vi "Rx Message to Transfer Handle - RT.vi"(8 "error in":errorcluster, 9 "message":T2={"name"="", "message type"="BC to RT", "endpoint Tx"={"terminal address"=0, "subaddress"=0}, "endpoint Rx"={"terminal address"=0, "subaddress"=0}, "create timestamp channel"=FALSE, "mode code"=0, "number of words"=0, "parameters"=[]}, 11 "remote terminal handles":u64[](array[numeric])) -> (0 "error out":errorcluster, 2 "valid?":bool, 3 "Rx read info":T1)   [LabVIEW 2020, in "AIM MIL-STD-1553 Engine.lvlib" / "Custom Device.lvlib"]
uses:
  Custom Device.lvlib
  Shared/Message Definition.ctl
  Shared/Message Type.ctl
  Shared/Terminal Endpoint.ctl
  Shared/Address.ctl
  Shared/Parameter Definition.ctl
  Shared/Rx Read Info.ctl
  <instrlib>/BTI1553Lib/Public/Controls/1553 Transfer Direction.ctl
  <instrlib>/BTI1553Lib/Public/Controls/1553 RT Transfer Type.ctl
  <instrlib>/BTI1553Lib/Private/RT/Configure/Get RT Xfer Handle.vi
  <instrlib>/BTI1553Lib/BTI1553LV.lvlib
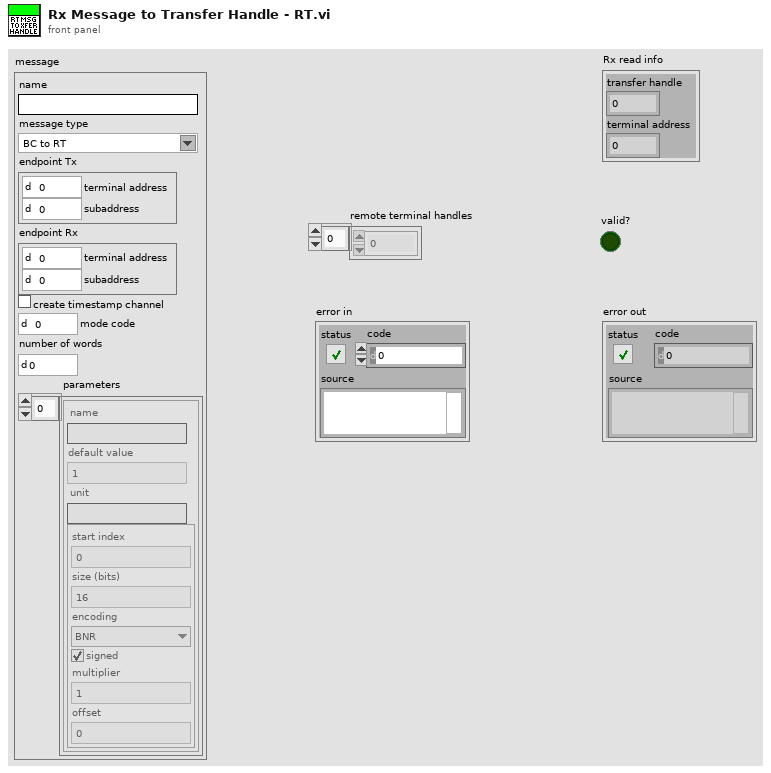
[diagram p1: front panel]
types:
  T1 = typedef "Rx Read Info.ctl" = cluster{"transfer handle":u64, "terminal address":u16}
  T2 = typedef "Message Definition.ctl" = cluster{"name":string, "message type":T3, "endpoint Tx":T4, "endpoint Rx":T4, "create timestamp channel":bool, "mode code":u16, "number of words":u16, "parameters":cluster{"name":string, "default value":dbl, "unit":string, "parameter definition":T6}[]}
  T3 = typedef "Message Type.ctl" = string
  T4 = typedef "Terminal Endpoint.ctl" = cluster{"terminal address":T5, "subaddress":T5}
  T5 = typedef "Address.ctl" = u16
  T6 = typedef "Parameter Definition.ctl" = cluster{"start index":i32, "size (bits)":i32, "encoding":enum16{"BNR", "BCD", "Discrete"}, "signed":bool, "multiplier":dbl, "offset":dbl}
  T7 = typedef "BTI1553LV.lvlib/1553 RT Transfer Type.ctl" = u32
  T8 = typedef "BTI1553LV.lvlib/1553 Transfer Direction.ctl" = u32
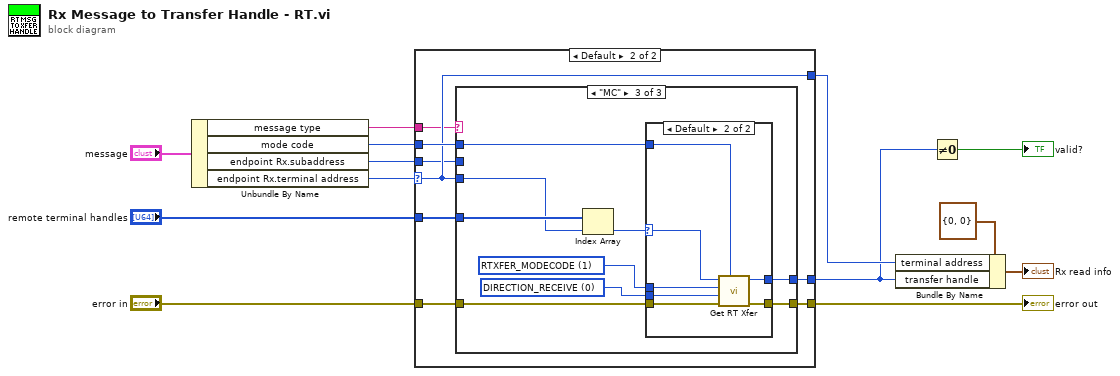
[diagram p0: block diagram]
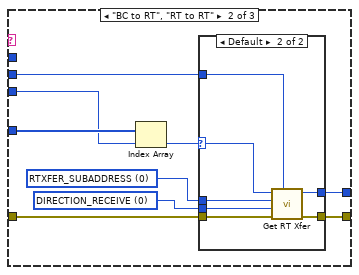
[diagram p4: hidden frame]
diagram:
  n1 = Unbundle By Name("message") -> ("message type"=w2:T3, "mode code"=w11:u16, "endpoint Rx.subaddress"=w1:T5, "endpoint Rx.terminal address"=w13:T5)
  n2 = case shown="Default" w13 {
    selector: w13 -> [_ w17]
    tunnel: "error in" -> [w14 w22]
    tunnel: [w14 w21] -> w8
    tunnel: "remote terminal handles" -> [_ w20]
    tunnel: w11 -> [_ w19]
    tunnel: [_ w18] -> w3
    tunnel: [_ w17] -> w5
    tunnel: w2 -> [_ w16]
    tunnel: w1 -> [_ w15]
    frame 0 {
    }
    frame Default {
      n3 = case shown="\"MC\"" w16 {
        tunnel: w22 -> [w23 w32 w49]
        tunnel: [w23 w31 w48] -> w21
        tunnel: w20 -> [_ w28 w45]
        tunnel: w19 -> [_ _ w43]
        tunnel: [_ w26 w42] -> w18
        tunnel: w17 -> [_ w25 w41]
        tunnel: w15 -> [_ w24 _]
        frame Default {
        }
        frame "BC to RT", "RT to RT" {
          w29 = T7 0 items=["RTXFER_SUBADDRESS", "RTXFER_MODECODE"] ("transfer type")
          w30 = T8 0 items=["DIRECTION_RECEIVE", "DIRECTION_TRANSMIT"] ("transfer direction")
          n4 = Index Array(array=w28, index=w25) -> (element=w27:u64)
          n5 = case shown="Default" w27 {
            selector: w27 -> [_ w36]
            tunnel: w32 -> [w33 w40]
            tunnel: [w33 w39] -> w31
            tunnel: w30 -> [_ w38]
            tunnel: w29 -> [_ w37]
            tunnel: [_ w35] -> w26
            tunnel: w24 -> [_ w34]
            frame 0, -1 {
            }
            frame Default {
              n6 = call-poly <instrlib>:"Get RT Xfer.vi"("transfer sa number or mc number"=w34, "error in (no error)"=w40, "transfer direction"=w38, "transfer type"=w37, "remote terminal handle in"=w36) -> ("error out"=w39:errorcluster, "rt transfer handle out"=w35:u64)  [unwired: 4 in, 1 out]
            }
          }
        }
        frame "MC" {
          w46 = T7 1 items=["RTXFER_SUBADDRESS", "RTXFER_MODECODE"] ("transfer type")
          w47 = T8 0 items=["DIRECTION_RECEIVE", "DIRECTION_TRANSMIT"] ("transfer direction")
          n7 = Index Array(array=w45, index=w41) -> (element=w44:u64)
          n8 = case shown="Default" w44 {
            selector: w44 -> [_ w53]
            tunnel: w49 -> [w50 w57]
            tunnel: [w50 w56] -> w48
            tunnel: w47 -> [_ w55]
            tunnel: w46 -> [_ w54]
            tunnel: w43 -> [_ w52]
            tunnel: [_ w51] -> w42
            frame 0, -1 {
            }
            frame Default {
              n9 = call-poly <instrlib>:"Get RT Xfer.vi"("transfer sa number or mc number"=w52, "error in (no error)"=w57, "transfer direction"=w55, "transfer type"=w54, "remote terminal handle in"=w53) -> ("error out"=w56:errorcluster, "rt transfer handle out"=w51:u64)  [unwired: 4 in, 1 out]
            }
          }
        }
      }
    }
  }
  "error out" <- w8
  n10 = Bundle By Name(cluster=T1 {"transfer handle"=0, "terminal address"=0} ("Rx read info"), "terminal address"=w5, "transfer handle"=w3) -> (→"Rx read info":T1)
  n11 = Not Equal To 0?(x=w3) -> (x != 0?=→"valid?":bool)
